vi "Point to Tree Item.vi"(8 "Error In":errorcluster, 10 "Coords":T1, 11 "reference":refnum<vi>) -> (0 "Error Out":errorcluster, 1 "In Bounds?":bool, 2 "Item":string, 4 "In Symbol?":bool, 5 "Valid":bool)   [LabVIEW 2016]
uses:
  <vilib>/Utility/miscctls.llb/LVPoint32TypeDef.ctl
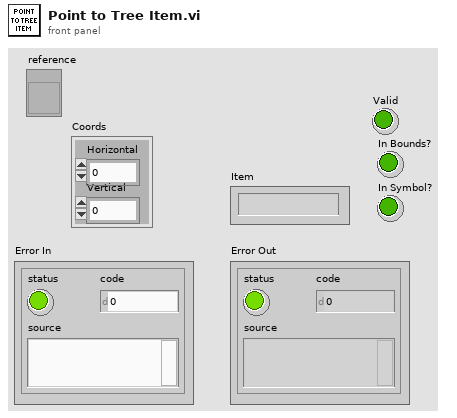
[diagram p1: front panel]
types:
  T1 = typedef "LVPoint32TypeDef.ctl" = cluster{"Horizontal":i32, "Vertical":i32}
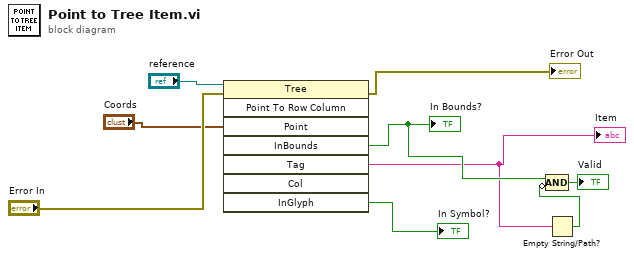
[diagram p0: block diagram]
diagram:
  n1 = invoke class="Tree" method="Point To Row Column"(reference="reference", error in="Error In", "Point"="Coords") -> (error out=→"Error Out":errorcluster, "InBounds"=w4:bool, "Tag"=w3:string, "InGlyph"=→"In Symbol?":bool)  [unwired: 5 in, 4 out]
  "Item" <- w3
  "In Bounds?" <- w4
  n2 = Empty String/Path?(string/path=w3) -> (empty?=w2:bool)
  n3 = Compound Arithmetic op=AND(w4, invert w2) -> (→"Valid":bool)
